vi "test drive.vi"() -> ()   [LabVIEW 2009]
uses:
  <vilib>/NXT/Subs/MotorOutput.ctl
  <vilib>/NXT/Subs/LVHSConnector.ctl
  <vilib>/NXT/Block Support/NXT_OutputPort.ctl
panel:
  in  "Connection":u16(ring) items=["USB", "Bluetooth", "USB then Bluetooth", "Last Connection", "Preference"]
  out "process variable":i32 caption="Position"
  in  "P coeffecient":sgl
  in  "stop":bool
  in  "Setpoint":i32(slide) scale=-100.0..0.0
  in  "Power":i8(slide)=75 scale=-100.0..100.0
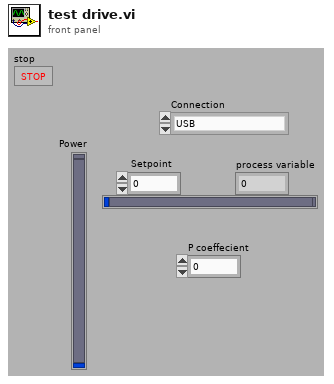
[diagram p1: front panel]
types:
  T1 = typedef "LVHSConnector.ctl" = cluster{"error":errorcluster, "address":string, "NXT #":i32, "Show Error":bool, "Connection":u16}
  T2 = typedef "MotorOutput.ctl" = u8
  T3 = typedef "NXT_OutputPort.ctl" = u8
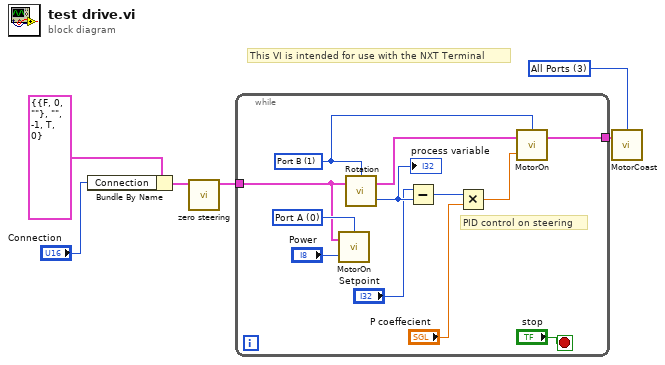
[diagram p0: block diagram]
diagram:
  w4 = T2 3 items=["Port A", "Port B", "Port C", "All Ports"] ("Port (All Ports)")
  # "This VI is intended for use with the NXT Terminal"
  n1 = Bundle By Name(cluster=T1 {"error"={"status"=FALSE, "code"=0, "source"=""}, "address"="", "NXT #"=-1, "Show Error"=TRUE, "Connection"=0} ("NXT"), "Connection"="Connection") -> (w2:T1)
  n2 = call "zero steering.vi"("NXT"=w2) -> ("NXT"=w6:T1)  [unwired: 10 in]
  n3 = while {
    tunnel: w6 -> [w14]
    tunnel: [w9] -> w5
    stop <- "stop" stop-if-true
    w8 = T3 1 items=["Port A", "Port B", "Port C"] ("Port (Port A)")
    w17 = T2 0 items=["Port A", "Port B", "Port C", "All Ports"] ("Output Port (All Ports)")
    # "PID control on steering"
    n4 = call <vilib>:"MotorOn.vi"("Power (75)"="Power", "NXT"=w14, "Output Port (All Ports)"=w17) -> ()  [unwired: 1 in, 1 out]
    n5 = call <vilib>:"Rotation.vi"("NXT"=w14, "Port (Port A)"=w8) -> ("Rotation"=w13:i32, "NXT"=w16:T1)  [unwired: 1 in]
    "process variable" <- w13
    n6 = Subtract(x="Setpoint", y=w13) -> (x-y=w12:i32)
    n7 = Multiply(x=w12, y="P coeffecient") -> (x*y=w10:sgl)
    n8 = call <vilib>:"MotorOn.vi"("Power (75)"=w10, "NXT"=w16, "Output Port (All Ports)"=w8) -> ("NXT"=w9:T1)  [unwired: 1 in]
  }
  n9 = call <vilib>:"MotorCoast.vi"("NXT"=w5, "Port (All Ports)"=w4) -> ()  [unwired: 2 in, 1 out]
